vi "最小频移键控MSK.vi"() -> ()   [LabVIEW 2015]
doc: "This example demonstrates the programming of an MSK Modulation Demodulation System."
uses:
  <vilib>/addons/Modulation/Digital/General/MT Generate Bits (Galois, PN Order).vi
  <vilib>/addons/Modulation/Digital/Support/Common/Validators/mod_Generate Bits Validate.vi
  <vilib>/addons/Modulation/Analog/support/mod_Set Error Source.vi
  <vilib>/addons/Modulation/Digital/Support/Common/Validators/mod_AWGN Validate.vi
  <vilib>/addons/Modulation/Digital/Impairments/subVIs/mod_createSeeds.vi
  <vilib>/addons/Modulation/Digital/Support/Common/Validators/mod_Validate Samples Per Symbol.vi
  <vilib>/addons/Modulation/Analog/support/Validators/mod_Validate Complex Waveform.vi
  <vilib>/addons/Modulation/Analog/support/Validators/mod_WFErrorHandler.vi
  <vilib>/addons/Modulation/Digital/Support/Common/Validators/mod_Generate Filter Coefficients Validate.vi
  <vilib>/addons/Modulation/Digital/General/subVIs/mod_Generate Filter Coefficients.vi
  <vilib>/addons/Modulation/Digital/General/subVIs/mod_Generate Bits PN Sequence.vi
  <vilib>/addons/Modulation/Digital/General/MT Generate MSK System Parameters.vi
  <vilib>/measure/maspectr.llb/FFT Spectrum (Mag-Phase) for 1 Chan.vi
  <vilib>/Analysis/1siggen.llb/Gaussian White Noise (obs 90).vi
  <vilib>/addons/Modulation/Digital/General/MT Apply Matched Filter (MSK).vi
  <vilib>/addons/Modulation/Digital/General/MT Align To Ideal Symbols (MSK).vi
  <vilib>/addons/Modulation/Digital/General/MT Map MSK Symbols to Bits.vi
  <vilib>/addons/Modulation/Digital/Demodulation/MT Calculate BER After Trigger (PN Sequence).vi
  <vilib>/addons/Modulation/niDMT.lvlib
  <vilib>/measure/NI_MAPro.lvlib
panel:
  out "input bit stream":i8[](array[numeric])
  in  "选项卡控件":enum32{"调制后时域", "调制后频谱", "星座图"}(tab)
  out "调制后时域":cluster{"f0":dbl, "df":dbl, "magnitude":dbl[]}(graph)
  out "调制后频谱":cluster{"f0":dbl, "df":dbl, "magnitude":dbl[]}(graph)
  out "星座图":T1(graph)
  in  "Eb/N0 (dB)":dbl(slide) scale=0.0..100.0
  in  "停止":bool
  out "复原消息位":i8[](array[numeric])
  in  "差分编码使能":enum16{"disable", "enable"}(ring)
  in  "种子":i32=-1
  out "error out":errorcluster
  out "误码率":dbl format="%.4f"
  in  "PN序列":i32=9
  in  "重置":bool=TRUE
  in  "符号速率(Hz)":dbl=400000.0 format="%.2p"
  in  "脉冲成形滤波器":T2(ring)=enum."Gaussian"
  in  "MSK符号":i32=1000
  in  "每符号采样数":i32=16
  # "最小频移键控MSK"
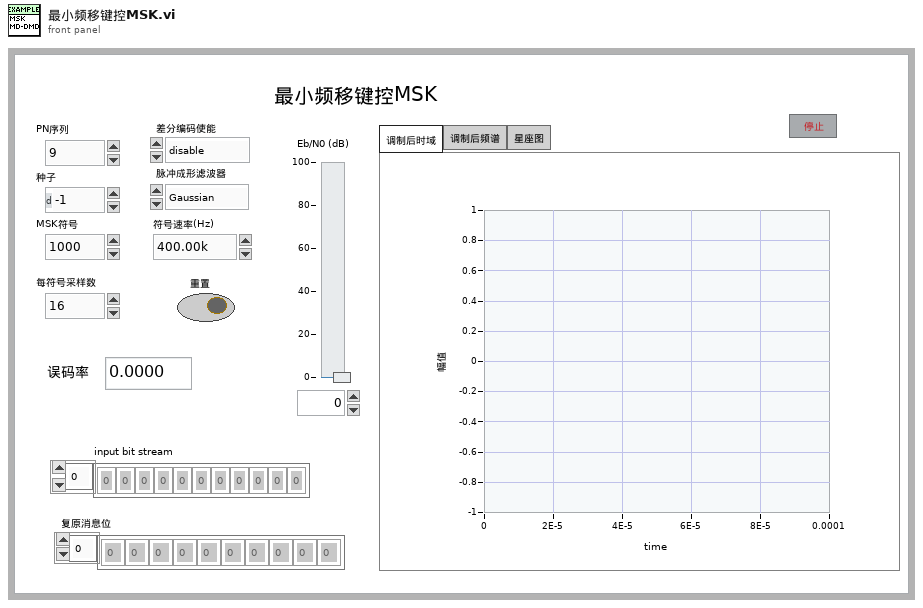
[diagram p1: front panel]
types:
  T1 = cluster{"constellation":dbl[], "oversampled data":dbl[]}[]
  T2 = enum16{"none", "Raised Cosine", "Root Raised Cos", "Gaussian"}
  T3 = enum16{"FSK", "PSK", "QAM", "MSK", "PAM", "ASK", "CPM"}
  T4 = cluster{"differential encoding enable":enum16{"disable", "enable"}, "samples per symbol (16)":i32}
  T5 = typedef "niAMT.lvlib/Complex Data Waveform.ctl" = cluster{"t0":dbl, "dt":dbl, "Y":cdb[]}
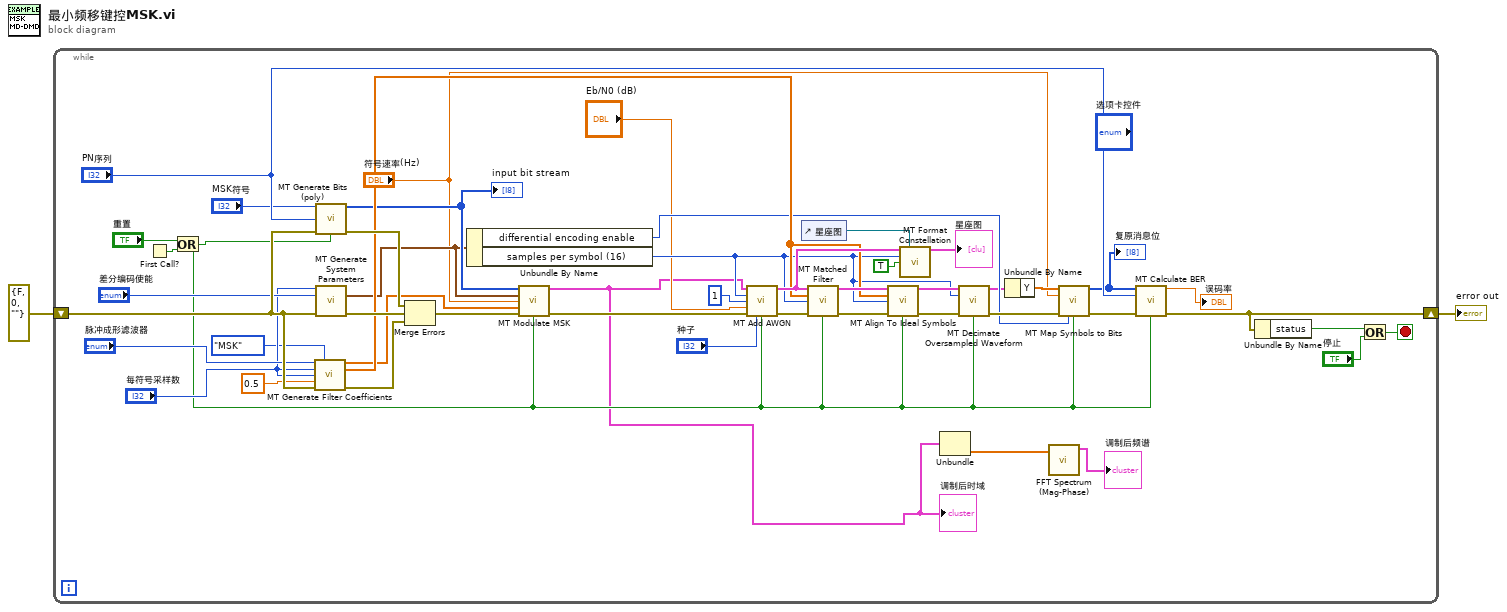
[diagram p0: block diagram]
diagram:
  n1 = while {
    shift-right: [w41] -> w2
    shift-left: errorcluster {"status"=FALSE, "code"=0, "source"=""} ("error out") -> [w50]
    stop <- w40 stop-if-true
    n2 = First Call?() -> (First Call?: T/F=w33:bool)
    n3 = Or(x="重置", y=w33) -> (x .or. y?=w14:bool)
    n4 = call <vilib>:"MT Generate Filter Coefficients.vi"("pulse shaping filter (none)"="脉冲成形滤波器", "modulation type"=T3."MSK", "pulse shaping samples per symbol (16)"="每符号采样数", "matched samples per symbol (16)"="每符号采样数", "filter parameter"=0.5, "error in (no error)"=w50) -> ("pulse shaping filter coefficients"=w7:dbl[], "matched filter coefficients"=w24:dbl[], "error out"=w45:errorcluster)  [unwired: 1 in, 6 out]
    n5 = call-poly <vilib>:"MT Generate Bits (poly).vi"("total bits (128)"="MSK符号", "PN sequence order (9)"="PN序列", "error in (no error)"=w50, "reset? (T)"=w14) -> ("output bit stream"=w17:i8[], "error out"=w47:errorcluster)  [unwired: 1 in, 9 out]
    "input bit stream" <- w17
    n6 = call-poly <vilib>:"MT Generate System Parameters.vi"("samples per symbol (16)"="每符号采样数", "differential encoding enable"="差分编码使能", "error in (no error)"=w50) -> ("MSK system parameters"=w16:T4, "error out"=w46:errorcluster)  [unwired: 2 in, 9 out]
    n7 = Merge Errors(w47, w46, w45) -> (w49:errorcluster)
    n8 = Unbundle By Name(w16) -> ("differential encoding enable"=w20:enum16{"disable", "enable"}, "samples per symbol (16)"=w18:i32)
    n9 = call <vilib>:"MT Modulate MSK.vi"("input bit stream"=w17, "MSK system parameters"=w16, "symbol rate (Hz)"="符号速率(Hz)", "pulse shaping filter coefficients"=w7, "error in (no error)"=w49, "reset? (T)"=w14) -> ("output complex waveform"=w6:T5, "error out"=w13:errorcluster)  [unwired: 1 in, 7 out]
    "调制后时域" <- w6
    n10 = call <vilib>:"MT Add AWGN.vi"("input complex waveform"=w6, "samples per symbol (16)"=w18, "bits per symbol (1)"=1, "Eb/N0 (10 dB)"="Eb/N0 (dB)", "error in (no error)"=w13, "seed in (0xFFFFFFFF)"="种子", "reset? (T)"=w14) -> ("output complex waveform"=w27:T5, "error out"=w32:errorcluster)  [unwired: 7 out]
    n11 = control-ref of="星座图"() -> (w10:refnum<vi>)
    n12 = call-poly <vilib>:"MT Matched Filter.vi"("input complex waveform"=w27, "matched filter coefficients"=w24, "samples per symbol (16)"=w18, "error in (no error)"=w32, "reset? (T)"=w14) -> ("output phase waveform"=w25:cluster{"t0":dbl, "dt":dbl, "Y":dbl[]}, "error out"=w28:errorcluster)  [unwired: 9 out]
    n13 = call-poly <vilib>:"MT Align To Ideal Symbols.vi"("input phase waveform"=w25, "matched filter coefficients"=w24, "samples per symbol (16)"=w18, "error in (no error)"=w28, "reset? (T)"=w14) -> ("output phase waveform"=w22:cluster{"t0":dbl, "dt":dbl, "Y":dbl[]}, "error out"=w26:errorcluster)  [unwired: 9 out]
    n14 = call <vilib>:"MT Format Constellation.vi"("waveform"=w27, "constellation reference"=w10, "samples per symbol"=w18, "autoscale"=TRUE) -> ("constellation graph"=→"星座图":T1)  [unwired: 1 in, 10 out]
    n15 = Unbundle(w6) -> ("Y"=w5:cdb[])  [unwired: 2 out]
    n16 = call <vilib>:"MT Decimate Oversampled Waveform.vi"("input complex waveform"=w22, "decimation factor"=w18, "error in (no error)"=w26, "reset? (T)"=w14) -> ("output complex waveform"=w3:T5, "error out"=w23:errorcluster)  [unwired: 1 in, 9 out]
    n17 = Unbundle By Name(w3) -> ("Y"=w21:cdb[])
    n18 = call-poly <vilib>:"FFT Spectrum (Mag-Phase).vi"("time signal"=w5) -> ("magnitude"=→"调制后频谱":cluster{"f0":dbl, "df":dbl, "magnitude":dbl[]})  [unwired: 6 in, 4 out]
    n19 = call-poly <vilib>:"MT Map Symbols to Bits.vi"("symbols"=w21, "symbol rate"="符号速率(Hz)", "error in (no error)"=w23, "differential encoding enable"=w20, "reset? (T)"=w14) -> ("output bit stream"=w30:i8[], "error out"=w29:errorcluster)  [unwired: 9 out]
    "复原消息位" <- w30
    n20 = call-poly <vilib>:"MT Calculate BER.vi"("input bit stream"=w30, "PN sequence order (9)"="PN序列", "error in (no error)"=w29, "reset? (T)"=w14) -> ("BER"=→"误码率":dbl, "error out"=w41:errorcluster)  [unwired: 2 in, 8 out]
    n21 = Unbundle By Name(w41) -> ("status"=w39:bool)
    n22 = Or(x=w39, y="停止") -> (x .or. y?=w40:bool)
  }
  "error out" <- w2
